vi "getAdditionalDataFromXMLNative.vi"(8 "error in (no error)":errorcluster, 10 "eventXML":refnum<k20>, 11 "SingleTone in":refnum<class "SingleTone.lvclass">) -> (0 "error out":errorcluster, 2 "eventXML out":refnum<k20>, 3 "SingleTone out":refnum<class "SingleTone.lvclass">)   [LabVIEW 2011, in "Tools.lvlib" / "Scripting.lvlib" / "SingleTone.lvclass"]
uses:
  SingleTone.lvclass
  SingleToneArray/SingleToneArray.lvclass
  SingleTone.lvclass/SingleTone.ctl
  <vilib>/xml/Close Reference(Node).vi
  <vilib>/xml/NI_XML.lvlib
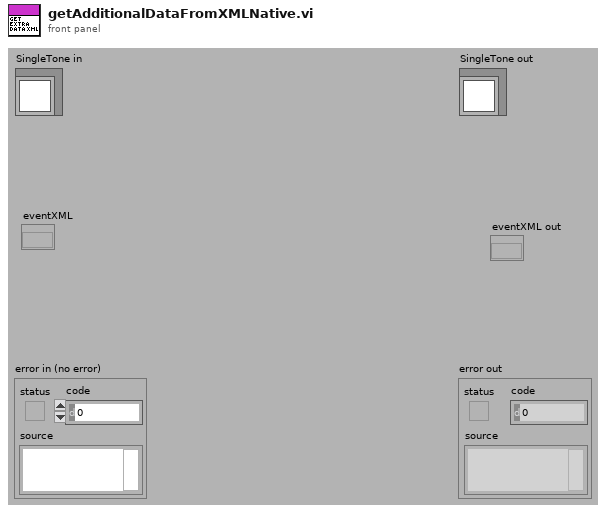
[diagram p1: front panel]
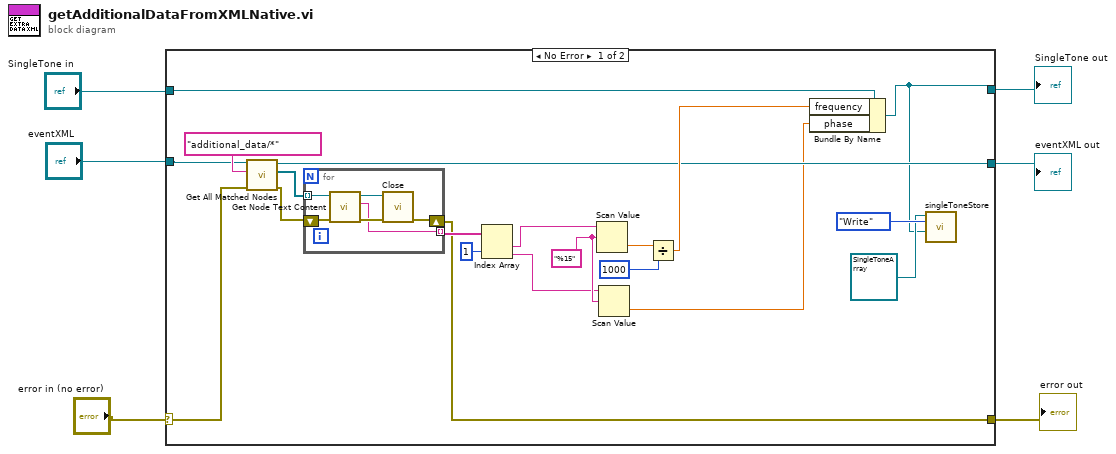
[diagram p0: block diagram]
diagram:
  n1 = case shown="No Error" "error in (no error)" {
    selector: "error in (no error)" -> [w16 w33]
    tunnel: [w7 w33] -> w1
    tunnel: "SingleTone in" -> [w23 w34]
    tunnel: [w8 w34] -> w3
    tunnel: [w15 _] -> w2
    tunnel: "eventXML" -> [w12 _]
    frame No Error {
      w22 = "%15"
      n2 = call <vilib>:"Get All Matched Nodes.vi"("error in (no error)"=w16, "XPath expression"="additional_data/*", "node in"=w12) -> ("error out"=w21:errorcluster, "node result array"=w19:refnum<k20>[], "node out"=w15:refnum<k20>)  [unwired: 6 in]
      n3 = for {
        tunnel: w19 -> [w29] mode=indexing
        tunnel: [w28] -> w18 mode=indexing
        shift-right: [w27] -> w7
        shift-left: w21 -> [w30]
        n4 = call <vilib>:"Get Node Text Content.vi"("error in (no error)"=w30, "node in"=w29) -> ("error out"=w31:errorcluster, "node text"=w28:string, "node out"=w32:refnum<k20>)  [unwired: 7 in]
        n5 = call-poly <vilib>:"Close.vi"("error in (no error)"=w31, "node"=w32) -> ("error out"=w27:errorcluster)  [unwired: 7 in]
      }
      n6 = Index Array(array=w18, index #2=1 ("index")) -> (element #1=w14:string, element #2=w13:string)  [unwired: 1 in]
      n7 = Scan Value(string=w14, format string=w22) -> (value=w26:dbl)  [unwired: 1 in, 1 out]
      n8 = Scan Value(string=w13, format string=w22) -> (value=w11:dbl)  [unwired: 1 in, 1 out]
      n9 = Divide(x=w26, y=1000) -> (x/y=w24:dbl)
      n10 = Bundle By Name(cluster=w23, "frequency"=w24, "phase"=w11) -> (w8:refnum<class "SingleTone.lvclass">)
      n11 = call "singleToneStore.vi"("SingleTone.lvclass"=w8, "action"=enum16{"Write", "Read"}."Write", "SingleToneArray in"=refnum<class "SingleToneArray.lvclass"> refnum) -> ()  [unwired: 5 in, 4 out]
    }
    frame Error {
    }
  }
  "error out" <- w1
  "SingleTone out" <- w3
  "eventXML out" <- w2
